vi "HiPOT Instrument UI.vi"() -> ()   [LabVIEW 2025, in "HiPOT.lvlib" / "HiPOT Instrument.lvclass"]
doc: "Copyright 2017 National Instruments Corporation\n\nLicensed under the Apache License, Version 2.0 (the \"License\"); you may not use this file except in compliance with the License. You may obtain a copy of the License at http://www.apache.org/licenses/LICENSE-2.0\nUnless required by applicable law or agreed to in writing, software distributed under the License is distributed on an \"AS IS\" BASIS, WITHOUT WARRANTIES OR CONDITIONS OF ANY KIND, either express or implied. See the License for the specific language governing permissions and limitations under the License."
uses:
  HiPOT Instrument.lvclass
  Users/Public/Documents/Sandia National Labs/TSS Plugin/CEF.lvlibp/Node/NodeRef.ctl
  Users/Public/Documents/Sandia National Labs/TSS Plugin/CEF.lvlibp/Node/CEF_Node.lvclass
  Users/Public/Documents/Sandia National Labs/TSS Plugin/CEF.lvlibp/Node/mainQref.ctl
  Users/Public/Documents/Sandia National Labs/TSS Plugin/CEF.lvlibp/Node/UserEventRef.ctl
  Users/Public/Documents/Sandia National Labs/TSS Plugin/Abstract Engine.lvlibp/Plugin/Abstract/Instrument configuration/Default Instrument.ctl
  HiPOT configuration/HiPOT Instrument Setting.ctl
  HiPOT Instrument.lvclass/HiPOT Instrument.ctl
  HiPOT configuration/HiPOT configuration.lvclass/HiPOT configuration.ctl
  HiPOT configuration/Read ACIR Setting.vi
  HiPOT configuration/Write ACIR Setting.vi
  <vilib>/Utility/error.llb/Trim Whitespace One-Sided.vi
  HiPOT configuration/HiPOT configuration.lvclass
  Users/Public/Documents/Sandia National Labs/TSS Plugin/Abstract Engine.lvlibp/Plugin/Abstract/Instrument configuration/Read Instrument Setting.vi
  Users/Public/Documents/Sandia National Labs/TSS Plugin/Abstract Engine.lvlibp/Plugin/Abstract/Instrument configuration/Write Instrument Setting.vi
  Users/Public/Documents/Sandia National Labs/TSS Plugin/Abstract Engine.lvlibp/Plugin/Abstract/Instrument configuration/Instrument configuration.lvclass
panel:
  in  "HiPOT":cluster{"Default":T1, "Setting":T2}={"Default"={"Type"="NI Digitizer", "Address"="None", "SW Alias"="None", "Description"="* Type = Class\n\n** Concrete = Specific  Device\nConcreate should be same with Type\n ", "Enabled"=TRUE}, "Setting"={"DC Voltage"=0.0, "High Limit"=100000.0, "Test Time(s)"=100000}} {"Setting"."High Limit" format="%#_6f"; "Setting"."DC Voltage" format="%#_6f"}
  in  "user event":T3
  in  "main queue":T4
  in  "node ref":T5
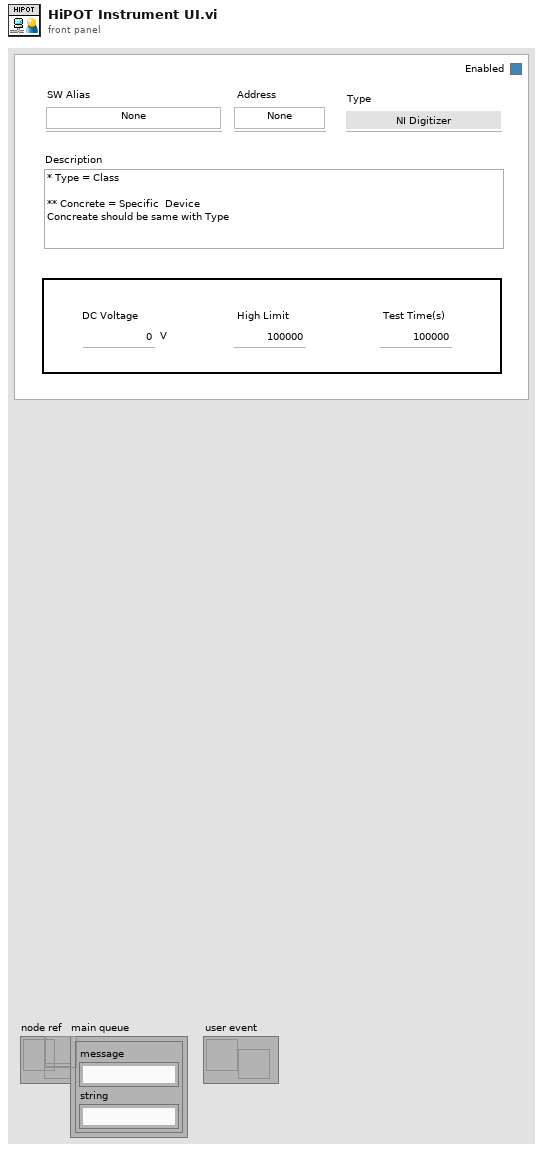
[diagram p1: front panel]
types:
  T1 = typedef "Abstract Engine.lvlibp/Instrument configuration.lvclass/Default Instrument.ctl" = cluster{"Type":string, "Address":string, "SW Alias":string, "Description":string, "Enabled":bool}
  T2 = typedef "HiPOT.lvlib/HiPOT configuration.lvclass/HiPOT Instrument Setting.ctl" = cluster{"DC Voltage":dbl, "High Limit":dbl, "Test Time(s)":u32}
  T3 = typedef "CEF.lvlibp/CEF_Node.lvclass/UserEventRef.ctl" = refnum<user-event>
  T4 = typedef "CEF.lvlibp/CEF_Node.lvclass/mainQref.ctl" = refnum<queue>
  T5 = typedef "CEF.lvlibp/CEF_Node.lvclass/NodeRef.ctl" = refnum<data-value>
  T6 = cluster{"Instrument Setting":T1, "HiPOT Setting":T2}
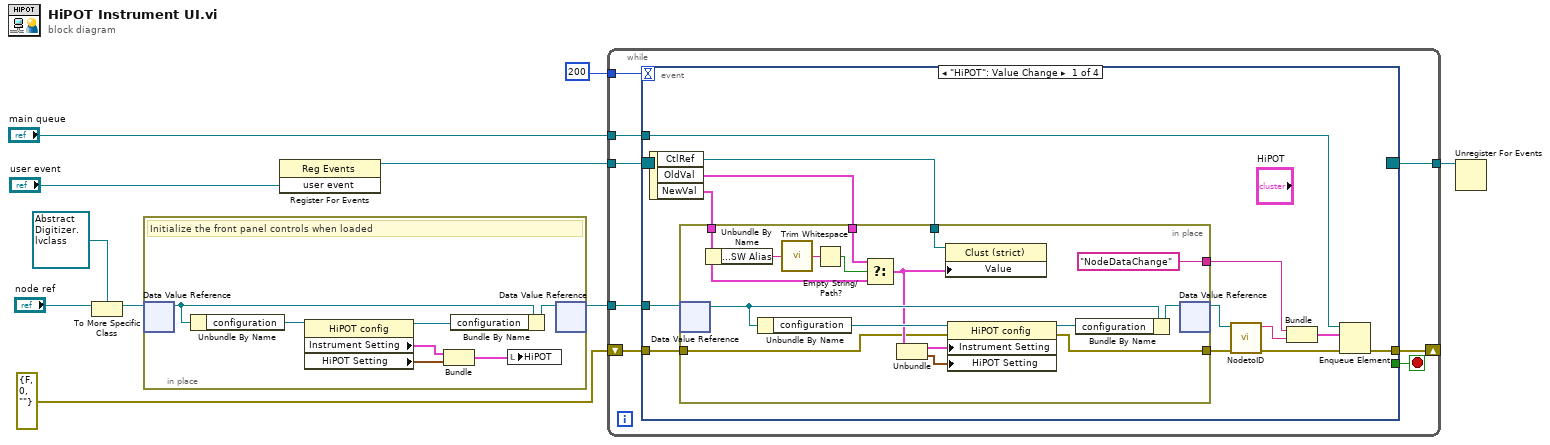
[diagram p0: block diagram]
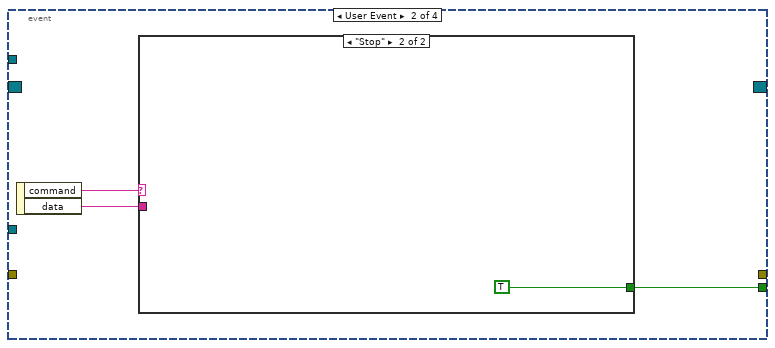
[diagram p2: hidden frame]
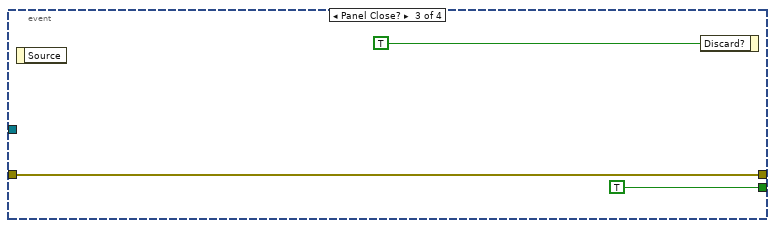
[diagram p4: hidden frame]
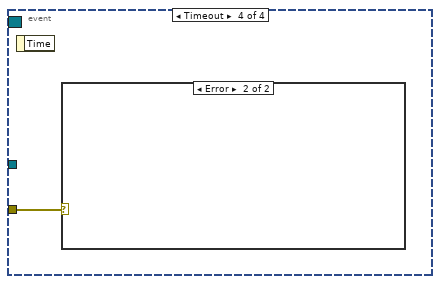
[diagram p5: hidden frame]
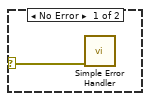
[diagram p6: hidden frame]
diagram:
  n1 = To More Specific Class(target class=refnum<data-value> refnum ("data value reference"), reference="node ref") -> (specific class reference=w2:refnum<data-value>)  [unwired: 1 in, 1 out]
  n2 = in-place {
    # "Initialize the front panel controls when loaded"
    n3 = in-place-dvr #1(w2) -> (w14:refnum<class "HiPOT Instrument.lvclass">)  [unwired: 1 out]
    n4 = Unbundle By Name(w14) -> ("configuration"=w15:refnum<class "HiPOT configuration.lvclass">)
    n5 = property class="HiPOT config"(reference=w15) -> (reference out=w13:refnum<class "HiPOT configuration.lvclass">, "Instrument Setting"=w12:T1, "HiPOT Setting"=w11:T2)  [unwired: 1 in, 1 out]
    n6 = Bundle("Instrument Setting"=w12, "HiPOT Setting"=w11) -> (w16:T6)  [unwired: 1 in]
    n7 = Bundle By Name(cluster=w14, "configuration"=w13) -> (w17:refnum<class "HiPOT Instrument.lvclass">)
    n8 = local write "HiPOT"(w16) -> ()
    n9 = in-place-dvr #1(w17) -> (w8:refnum<data-value>)  [unwired: 1 out]
  }
  n10 = register-events("user event") -> (reference out=w5:refnum<event-registration>)  [unwired: 2 in, 1 out]
  n11 = while {
    tunnel: w8 -> [w25]
    tunnel: "main queue" -> [w22]
    tunnel: 200 -> [w20]
    tunnel: [w21] -> w6
    tunnel: w5 -> [w19]
    shift-right: [w23] -> _
    shift-left: errorcluster {"status"=FALSE, "code"=0, "source"=""} ("error out") -> [w18]
    stop <- w24 stop-if-true
    n12 = event shown="[0] \"HiPOT\": Value Change" {
      selector: w19 -> [_ _ _ _]
      dyn-events: [_ _ _ _] -> w21
      timeout: w20 -> [_ _ _ _]
      tunnel: w25 -> [w36 _ _ _]
      tunnel: [_ w55 TRUE _] -> w24
      tunnel: [w38 _ w59 _] -> w23
      tunnel: w22 -> [w37 _ _ _]
      tunnel: w18 -> [w31 _ w59 w62]
      event "HiPOT": Value Change {
        n13 = event-data() -> ("CtlRef"=w33:refnum<vi>, "OldVal"=w34:cluster{"Default":T1, "Setting":T2}, "NewVal"=w32:cluster{"Default":T1, "Setting":T2})  [unwired: 1 in]
        n14 = in-place {
          in-place-border: [w51] -> w27
          in-place-border: w34 -> [w50]
          in-place-border: w33 -> [w49]
          in-place-border: w32 -> [w46]
          in-place-border: w31 -> [w40]
          in-place-border: ["NodeDataChange" ("Message Name")] -> w30
          n15 = in-place-dvr #2(w36) -> (w54:refnum<class "HiPOT Instrument.lvclass">)  [unwired: 1 out]
          n16 = Unbundle By Name(w46) -> ("Default.SW Alias"=w48:string)
          n17 = Unbundle By Name(w54) -> ("configuration"=w44:refnum<class "HiPOT configuration.lvclass">)
          n18 = call <vilib>:"Trim Whitespace.vi"("string"=w48) -> ("trimmed string"=w45:string)  [unwired: 1 in]
          n19 = Empty String/Path?(string/path=w45) -> (empty?=w47:bool)
          n20 = Select(t=w50, s=w47, f=w46) -> (s? t:f=w43:cluster{"Default":T1, "Setting":T2})
          n21 = Unbundle(w43) -> ("Default"=w42:T1, "Setting"=w41:T2)
          n22 = property class="Clust (strict)"(reference=w49, "Value"=w43) -> ()  [unwired: 1 in, 2 out]
          n23 = property class="HiPOT config"(reference=w44, error in=w40, "Instrument Setting"=w42, "HiPOT Setting"=w41) -> (reference out=w52:refnum<class "HiPOT configuration.lvclass">, error out=w51:errorcluster)
          n24 = Bundle By Name(cluster=w54, "configuration"=w52) -> (w53:refnum<class "HiPOT Instrument.lvclass">)
          n25 = in-place-dvr #2(w53) -> (w35:refnum<data-value>)  [unwired: 1 out]
        }
        n26 = call "NodetoID.vi"("error in"=w27, "node ref"=w35) -> ("error out"=w26:errorcluster, "ID"=w29:string)  [unwired: 8 in]
        n27 = Bundle("Message Name"=w30, "ID"=w29) -> (w28:cluster{"Message Name":string, "ID":string})  [unwired: 1 in]
        n28 = Enqueue Element(queue=w37, element=w28, error in (no error)=w26) -> (error out=w38:errorcluster)  [unwired: 1 in, 2 out]
      }
      event User Event {
        n29 = event-data() -> ("command"=w57:string, "data"=w56:string)  [unwired: 1 in]
        n30 = case shown="\"Stop\"" w57 {
          tunnel: w56 -> [_ _]
          tunnel: [_ TRUE] -> w55
          frame Default {
          }
          frame "Stop" {
          }
        }
      }
      event Panel Close? {
        n31 = event-data() -> ()  [unwired: 1 in, 1 out]
        n32 = event-data("Discard?"=TRUE) -> ()  [unwired: 1 in, 1 out]
      }
      event Timeout {
        n33 = event-data() -> ()  [unwired: 1 in, 1 out]
        n34 = case shown="Error" w62 {
          selector: w62 -> [w63 _]
          frame No Error {
            n35 = call <vilib>:"Simple Error Handler.vi"("error in (no error)"=w63) -> ()  [unwired: 4 in, 5 out]
          }
          frame Error {
          }
        }
      }
    }
  }
  n36 = Unregister For Events(event registration refnum=w6) -> ()  [unwired: 1 in, 1 out]
